vi "Empty Channel Settings.vi"() -> (0 "Channel Settings":T1={"Name"="", "Terminal Information"={"IO Device"=enum."none", "Channel Number"=0}, "Calibration Information"={"Excitation Voltage"=0.0, "Calibration Factor"=0.0, "Zero Value"=0.0, "Calibration Formula"="(x-x0) / (Ve * CF)"}})   [LabVIEW 2021, in "Acquisition.lvlib"]
doc: "(inline VI) Return an empty Channel Settings value. Use in-place of a block diagram constant."
uses:
  Acquisition.lvlib
  IO Device.ctl
  Channel Settings.ctl
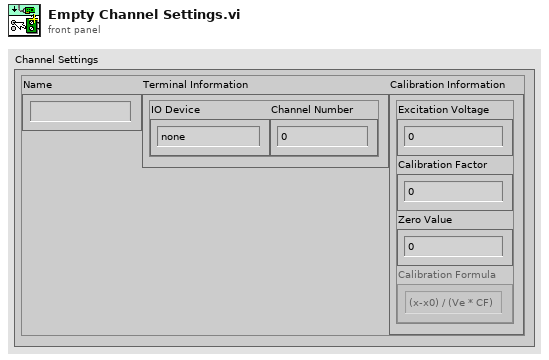
[diagram p1: front panel]
types:
  T1 = typedef "Acquisition.lvlib/Channel Settings.ctl" = cluster{"Name":string, "Terminal Information":cluster{"IO Device":T2, "Channel Number":i32}, "Calibration Information":cluster{"Excitation Voltage":dbl, "Calibration Factor":dbl, "Zero Value":dbl, "Calibration Formula":string}}
  T2 = typedef "Acquisition.lvlib/IO Device.ctl" = enum16{"none", "9219", "9401"}
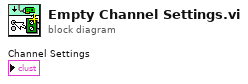
[diagram p0: block diagram]
diagram:
